vi "range.vi"() -> ()   [LabVIEW 2021]
uses:
  <vilib>/Instr/_visa.llb/VISA Configure Serial Port (Instr).vi
panel:
  in  "stop":bool
  in  "VISA resource name":refnum<visa-resource-name>="COM7"
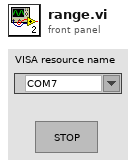
[diagram p1: front panel]
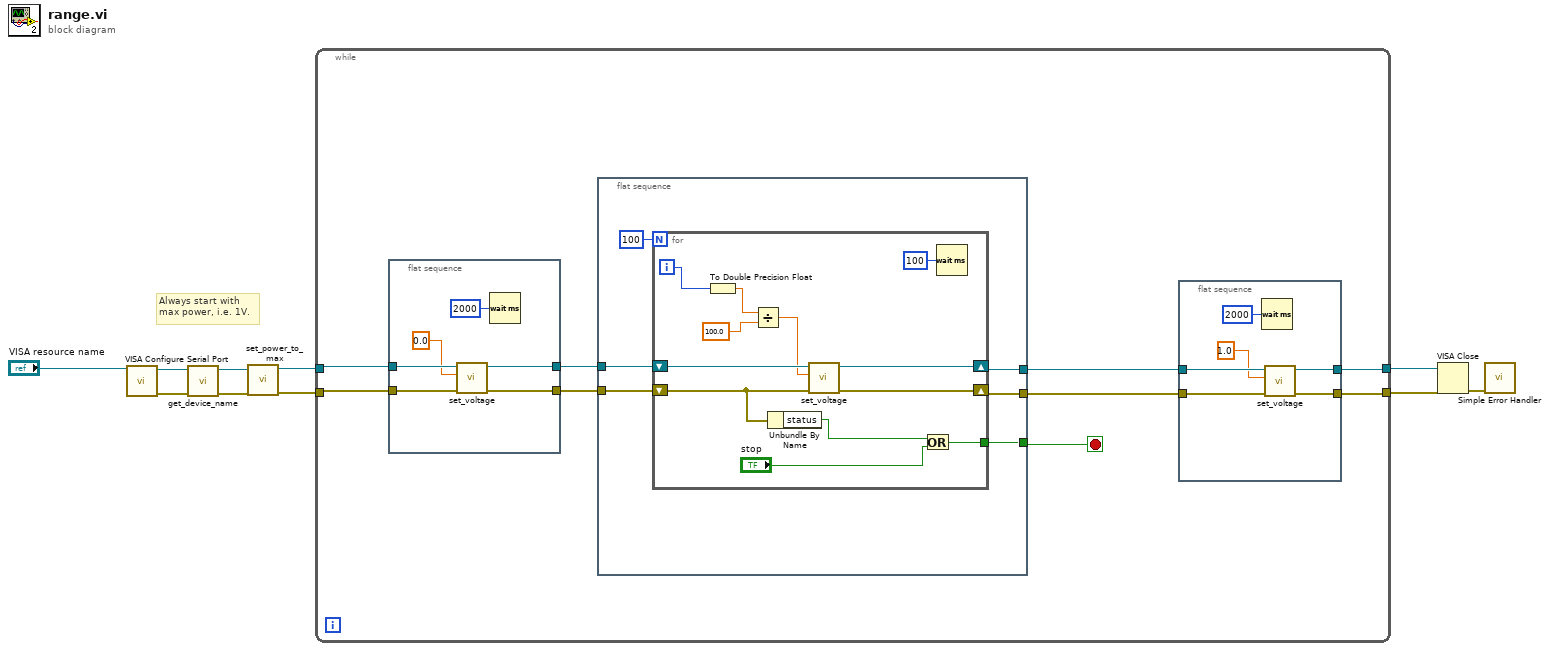
[diagram p0: block diagram]
diagram:
  # "Always start with\nmax power, i.e. 1V."
  n1 = call-poly "VISA Configure Serial Port"("VISA resource name"="VISA resource name") -> ("VISA resource name out"=w3:refnum<visa-resource-name>, "error out"=w4:errorcluster)  [unwired: 9 in, 4 out]
  n2 = call "get_device_name.vi"("error in"=w4, "VISA resource name in"=w3) -> ("error out"=w5:errorcluster, "VISA resource name out"=w6:refnum<visa-resource-name>)  [unwired: 7 in, 1 out]
  n3 = call "set_power_to_max.vi"("error in"=w5, "VISA resource name"=w6) -> ("error out"=w1:errorcluster, "VISA resource name out"=w2:refnum<visa-resource-name>)  [unwired: 8 in]
  n4 = while {
    tunnel: [w11] -> w8
    tunnel: [w12] -> w7
    tunnel: w2 -> [w18]
    tunnel: w1 -> [w17]
    stop <- w19 stop-if-true
    n5 = flat-sequence {
      tunnel: w18 -> [w49]
      tunnel: w17 -> [w48]
      tunnel: [w46] -> w16
      tunnel: [w45] -> w15
      frame #0 {
        n6 = call "set_voltage.vi"("error in"=w48, "voltage"=0.0, "VISA resource name"=w49) -> ("error out"=w45:errorcluster, "VISA resource name out"=w46:refnum<visa-resource-name>)  [unwired: 6 in, 1 out]
        n7 = Wait (ms)(milliseconds to wait=u32 2000) -> ()  [unwired: 1 out]
      }
    }
    n8 = flat-sequence {
      tunnel: [w31] -> w19
      tunnel: w16 -> [w30]
      tunnel: w15 -> [w29]
      tunnel: [w27] -> w14
      tunnel: [w26] -> w13
      frame #0 {
        n9 = for {
          N: 100 -> [_]
          shift-right: [w43] -> w27
          shift-left: w30 -> [w41]
          shift-right: [w42] -> w26
          shift-left: w29 -> [w39]
          tunnel: [w36] -> w31
          i -> [w35]
          n10 = To Double Precision Float(number=w35) -> (double precision float=w34:dbl)
          n11 = Divide(x=w34, y=100.0) -> (x/y=w32:dbl)
          n12 = Unbundle By Name(w39) -> ("status"=w37:bool)
          n13 = call "set_voltage.vi"("error in"=w39, "voltage"=w32, "VISA resource name"=w41) -> ("error out"=w42:errorcluster, "VISA resource name out"=w43:refnum<visa-resource-name>)  [unwired: 6 in, 1 out]
          n14 = Or(x=w37, y="stop") -> (x .or. y?=w36:bool)
          n15 = Wait (ms)(milliseconds to wait=u32 100) -> ()  [unwired: 1 out]
        }
      }
    }
    n16 = flat-sequence {
      tunnel: w14 -> [w25]
      tunnel: w13 -> [w24]
      tunnel: [w23] -> w12
      tunnel: [w22] -> w11
      frame #0 {
        n17 = Wait (ms)(milliseconds to wait=u32 2000) -> ()  [unwired: 1 out]
        n18 = call "set_voltage.vi"("error in"=w24, "voltage"=1.0, "VISA resource name"=w25) -> ("error out"=w22:errorcluster, "VISA resource name out"=w23:refnum<visa-resource-name>)  [unwired: 6 in, 1 out]
      }
    }
  }
  n19 = VISA Close(VISA resource name=w7, error in (no error)=w8) -> (error out=w9:errorcluster)
  n20 = call <vilib>:"Simple Error Handler.vi"("error in (no error)"=w9) -> ()  [unwired: 1 in, 8 out]
